vi "BPSK_tx.vi"() -> ()   [LabVIEW 2022 SP3]
uses:
  <instrlib>/niUSRP/niUSRP Write Tx Data (CDB WDT).vi
  <vilib>/Analysis/NI_AALPro.lvlib
  <vilib>/Analysis/NI_AALBase.lvlib
panel:
  in  "active antenna":string
  out "Waveform Chart 2":dbl[](graph)
  out "Array":dbl[](array[numeric])
  out "input array":dbl[](array[numeric])
  in  "standard deviation":dbl=1.0000000000000002 format="%0.2f"
  in  "No.of bits take 10":i32
  out "Waveform Chart":dynamicdata(graph)
  in  "gain 2":dbl format="%#_6f"
  in  "carrier frequency 2":dbl=100000.0 format="%#_6p"
  in  "IQ rate 2":dbl=100000.0 format="%#_6p"
  in  "device names 2":refnum<k15>
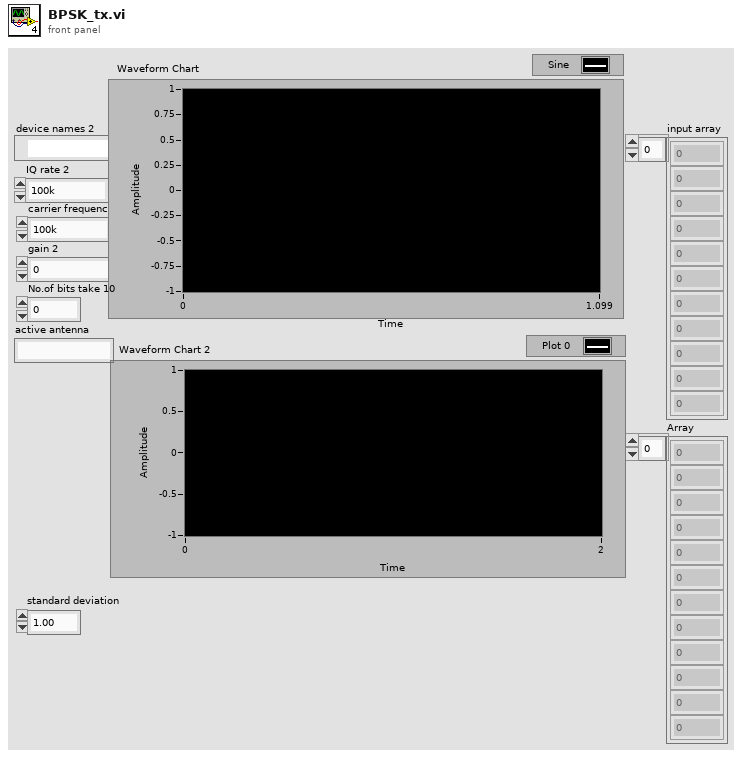
[diagram p1: front panel]
types:
  T1 = enum16{"sine", "cosine", "triangle", "square", "sawtooth", "increasing ramp", "decreasing ramp"}
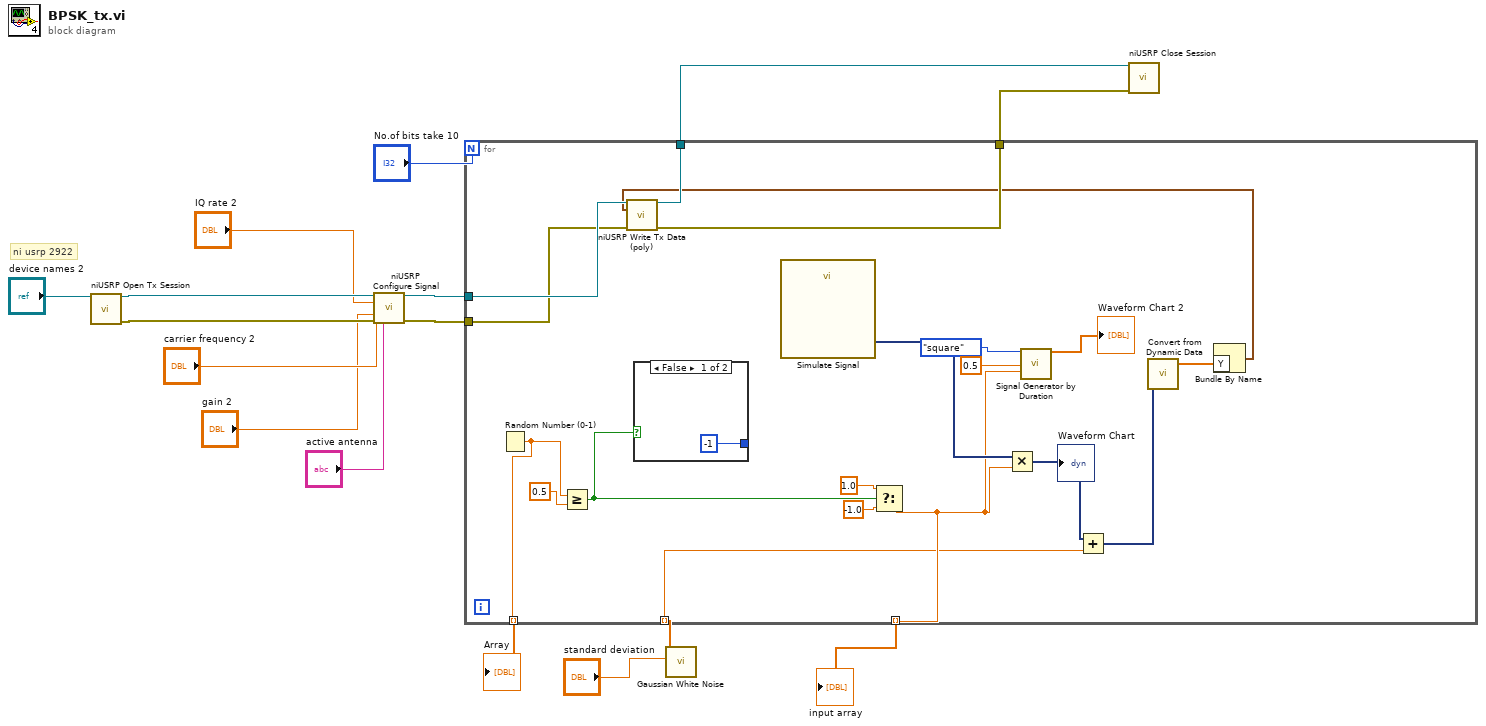
[diagram p0: block diagram]
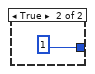
[diagram p2: hidden frame]
diagram:
  # "ni usrp 2922"
  n1 = call <instrlib>:"niUSRP Open Tx Session.vi"("device names"="device names 2") -> ("session handle out"=w15:refnum<k15>, "error out"=w14:errorcluster)  [unwired: 13 in]
  n2 = call <instrlib>:"niUSRP Configure Signal.vi"("session handle"=w15, "IQ rate"="IQ rate 2", "carrier frequency"="carrier frequency 2", "gain"="gain 2", "error in (no error)"=w14, "active antenna"="active antenna") -> ("session handle out"=w5:refnum<k15>, "error out"=w4:errorcluster)  [unwired: 5 in, 3 out]
  n3 = call <vilib>:"Gaussian White Noise.vi"("standard deviation"="standard deviation") -> ("Gaussian noise pattern"=w8:dbl[])  [unwired: 9 in, 1 out]
  n4 = for {
    N: "No.of bits take 10" -> [_]
    tunnel: w8 -> [w18] mode=indexing
    tunnel: [w27] -> w7 mode=indexing
    tunnel: [w26] -> w6 mode=indexing
    tunnel: w5 -> [w25]
    tunnel: w4 -> [w24]
    tunnel: [w23] -> w3
    tunnel: [w22] -> w2
    n5 = Random Number (0-1)() -> (number: 0 to 1=w26:dbl)
    n6 = Greater Or Equal?(x=w26, y=0.5) -> (x >= y?=w32:bool)
    n7 = case shown="False" w32 {
      tunnel: [-1 1] -> _
      frame False {
      }
      frame True {
      }
    }
    n8 = call "Simulate Signal"() -> ("Sine"=w31:dynamicdata)  [unwired: 14 in, 1 out]
    n9 = Select(t=1.0, s=w32, f=-1.0) -> (s? t:f=w27:dbl)
    n10 = Multiply(x=w31, y=w27) -> (x*y=w28:dynamicdata)
    "Waveform Chart" <- w28
    n11 = call <vilib>:"Signal Generator by Duration.vi"("signal type"=T1."square", "frequency"=0.5, "amplitude"=w27) -> ("signal"=→"Waveform Chart 2":dbl[])  [unwired: 9 in, 3 out]
    n12 = Add(x=w28, y=w18) -> (x+y=w21:dynamicdata)
    n13 = call "Convert from Dynamic Data"("Dynamic Data Type"=w21) -> ("Array"=w20:dbl[])  [unwired: 3 in]
    n14 = Bundle By Name("Y"=w20) -> (w17:waveform(dbl))  [unwired: 1 in]
    n15 = call-poly <instrlib>:"niUSRP Write Tx Data (poly).vi"("session handle"=w25, "data"=w17, "error in (no error)"=w24) -> ("session handle out"=w23:refnum<k15>, "error out"=w22:errorcluster)  [unwired: 11 in]
  }
  "input array" <- w7
  "Array" <- w6
  n16 = call <instrlib>:"niUSRP Close Session.vi"("session handle"=w3, "error in (no error)"=w2) -> ()  [unwired: 13 in, 1 out]
